vi "子VI-工件信息输入.vi"(8 "Y Resolution":i32, 9 "X Resolution":i32) -> (0 "质量等级":string, 1 "模式选择":u16(ring) items=["只读穿透图", "穿透图和反射图结合"], 2 "框号字体大小-":i16, 3 "产品规格":cluster{"产品长度（周长）（mm）":dbl, "产品宽度（母线长）（mm）":dbl}, 4 "是否需要预处理":u16, 5 "图像分辨率":T1)   [LabVIEW 2018]
panel:
  in  "框号字体大小":i16
  in  "是否需要预处理（默认不进行预处理）":u16(ring) items=["需要预处理", "不需要预处理"]
  in  "模式选择":u16(ring) items=["只读穿透图", "穿透图和反射图结合"]
  in  "质量等级（请填入A/B/C，默认为B）":u16(ring) items=["A", "B", "C"]
  out "错误常量out":errorcluster
  in  "错误常量":errorcluster
  in  "停止按钮":bool
  in  "产品宽度（母线长）（mm）":dbl format="%#_13g"
  in  "产品长度（周长）（mm）":dbl format="%#_13g"
  in  "图像Y向分辨率（mm/像素）":dbl=1.0 format="%#_13g"
  in  "图像X向分辨率（mm/像素）":dbl=1.0 format="%#_13g"
  # "图像及工件参数输入"
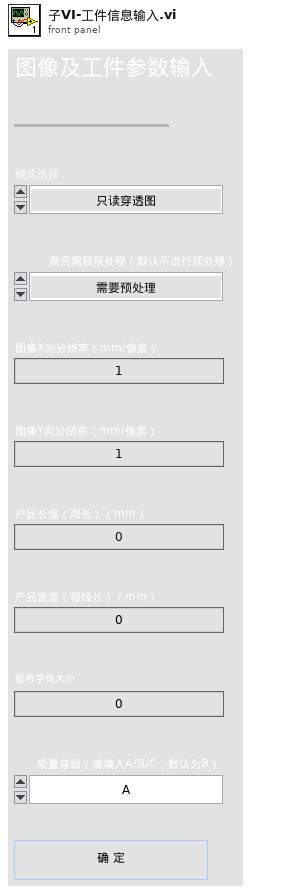
[diagram p1: front panel]
types:
  T1 = cluster{"图像X向分辨率（mm/像素）":dbl, "图像Y向分辨率（mm/像素）":dbl}
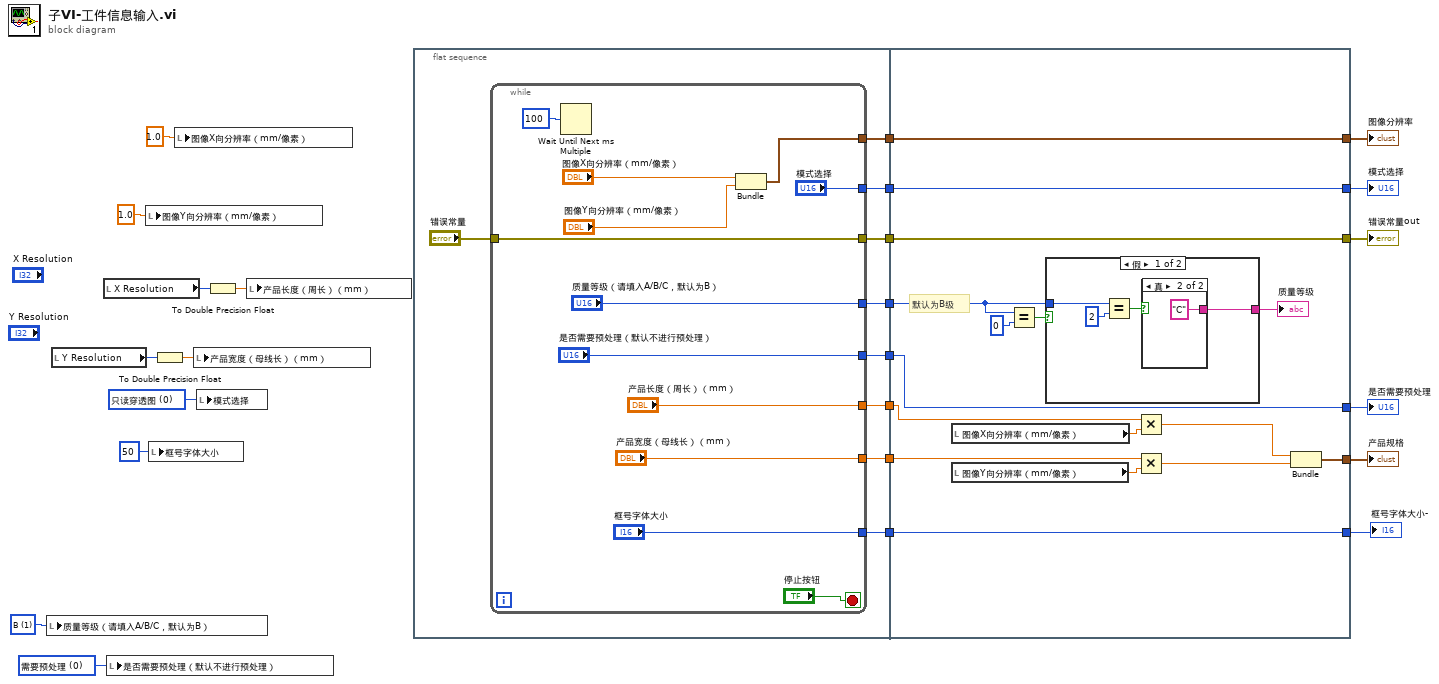
[diagram p0: block diagram]
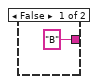
[diagram p2: hidden frame]
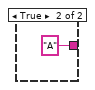
[diagram p3: hidden frame]
diagram:
  w12 = u16 0 items=["需要预处理", "不需要预处理"] ("是否需要预处理（默认不进行预处理）")
  w19 = u16 1 items=["A", "B", "C"] ("质量等级（请填入A/B/C，默认为B）")
  w20 = u16 0 items=["只读穿透图", "穿透图和反射图结合"] ("模式选择（默认只读穿透图）")
  n1 = local write "质量等级（请填入A/B/C，默认为B）"(w19) -> ()
  n2 = local read "Y Resolution"() -> (w16:i32)
  n3 = local read "X Resolution"() -> (w18:i32)
  n4 = local write "是否需要预处理（默认不进行预处理）"(w12) -> ()
  n5 = local write "图像Y向分辨率（mm/像素）"(1.0 ("图像Y向分辨率（mm/像素）")) -> ()
  n6 = local write "框号字体大小"(i8 50 ("框号字体大小")) -> ()
  n7 = To Double Precision Float(number=w16) -> (double precision float=w15:dbl)
  n8 = local write "图像X向分辨率（mm/像素）"(1.0 ("图像X向分辨率（mm/像素）")) -> ()
  n9 = local write "产品宽度（母线长）（mm）"(w15) -> ()
  n10 = local write "模式选择"(w20) -> ()
  n11 = To Double Precision Float(number=w18) -> (double precision float=w17:dbl)
  n12 = local write "产品长度（周长）（mm）"(w17) -> ()
  n13 = flat-sequence {
    tunnel: [w33] -> w11
    tunnel: [w32] -> w10
    tunnel: [w31] -> w9
    tunnel: [w30] -> w8
    tunnel: [w28] -> w7
    tunnel: [w27] -> w5
    tunnel: [w26] -> w4
    tunnel: [w25] -> w2
    tunnel: [w59] -> w21
    tunnel: [w60] -> w22
    tunnel: [w53] -> w23
    tunnel: [w61] -> w24
    tunnel: w11 -> [w61]
    tunnel: w10 -> [w60]
    tunnel: w9 -> [w59]
    tunnel: w8 -> [w56]
    tunnel: w7 -> [w54]
    tunnel: [w54] -> w6
    tunnel: w5 -> [w52]
    tunnel: w4 -> [w48]
    tunnel: [w46] -> w1
    tunnel: w2 -> [w46]
    frame #0 {
      n14 = while {
        tunnel: [w45] -> w33
        tunnel: "错误常量" -> [w41]
        tunnel: [w41] -> w32
        tunnel: ["质量等级（请填入A/B/C，默认为B）"] -> w30
        tunnel: ["模式选择"] -> w31
        tunnel: ["是否需要预处理（默认不进行预处理）"] -> w28
        tunnel: ["产品长度（周长）（mm）"] -> w27
        tunnel: ["产品宽度（母线长）（mm）"] -> w26
        tunnel: ["框号字体大小"] -> w25
        stop <- "停止按钮" stop-if-true
        n15 = Wait Until Next ms Multiple(millisecond multiple=u32 100 ("毫秒倍数")) -> ()  [unwired: 1 out]
        n16 = Bundle("图像X向分辨率（mm/像素）"="图像X向分辨率（mm/像素）", "图像Y向分辨率（mm/像素）"="图像Y向分辨率（mm/像素）") -> (w45:T1)  [unwired: 1 in]
      }
    }
    frame #1 {
      # "默认为B级"
      n17 = local read "图像X向分辨率（mm/像素）"() -> (w51:dbl)
      n18 = local read "图像Y向分辨率（mm/像素）"() -> (w47:dbl)
      n19 = Equal?(x=w56, y=u16 0) -> (x = y?=w57:bool)
      n20 = case shown="假" w57 {
        tunnel: [w62 "A" ("质量等级")] -> w58
        tunnel: w56 -> [w64 _]
        frame False {
          n21 = Equal?(x=w64, y=u16 2) -> (x = y?=w63:bool)
          n22 = case shown="真" w63 {
            tunnel: ["B" ("质量等级") "C" ("质量等级")] -> w62
            frame False {
            }
            frame True {
            }
          }
        }
        frame True {
        }
      }
      "质量等级" <- w58
      n23 = Multiply(x=w52, y=w51) -> (x*y=w50:dbl)
      n24 = Multiply(x=w48, y=w47) -> (x*y=w49:dbl)
      n25 = Bundle(w50, w49) -> (w53:cluster{dbl, dbl})  [unwired: 1 in]
    }
  }
  "图像分辨率" <- w24
  "产品规格" <- w23
  "错误常量out" <- w22
  "模式选择" <- w21
  "是否需要预处理" <- w6
  "框号字体大小-" <- w1
